vi "Write Camera Type.vi"(8 "error in (no error)":errorcluster, 10 "Camera Type":T1, 11 "Virtual Camera in":refnum<class "Virtual Camera.lvclass">) -> (0 "error out":errorcluster, 3 "Virtual Camera out":refnum<class "Virtual Camera.lvclass">)   [LabVIEW 2015]
uses:
  Virtual Camera.lvclass
  Resources/Type Defs/Camera Type.ctl
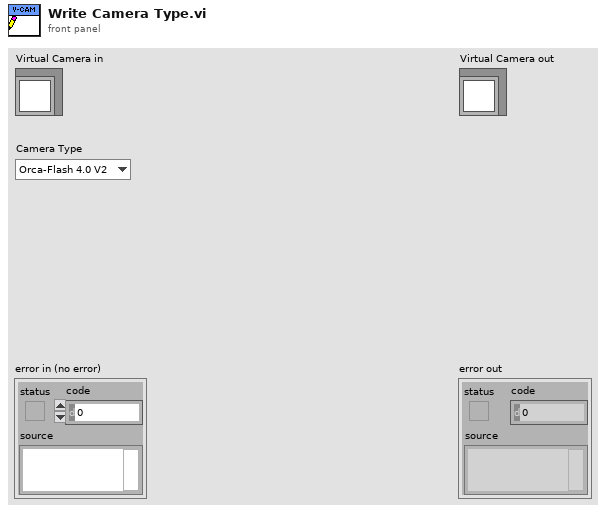
[diagram p1: front panel]
types:
  T1 = typedef "Camera Type.ctl" = enum16{"Orca-Flash 4.0 V2"}
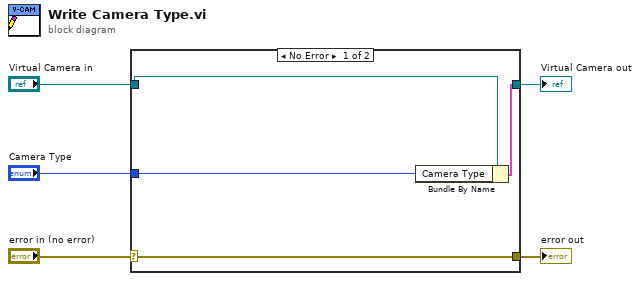
[diagram p0: block diagram]
diagram:
  n1 = case shown="No Error" "error in (no error)" {
    selector: "error in (no error)" -> [w9 w10]
    tunnel: [w9 w10] -> w4
    tunnel: [w7 w11] -> w2
    tunnel: "Virtual Camera in" -> [w8 w11]
    tunnel: "Camera Type" -> [w6 _]
    frame No Error {
      n2 = Bundle By Name(cluster=w8, "Camera Type"=w6) -> (w7:cluster{})
    }
    frame Error {
    }
  }
  "error out" <- w4
  "Virtual Camera out" <- w2
